vi "Write TDMS File.vi"(6 "Data Array":dbl[](array[numeric]), 8 "error in":errorcluster, 9 "Data & Time String":string, 10 "Header":string, 11 "Path":path) -> (0 "error out":errorcluster)   [LabVIEW 2009]
doc: "This subVI writes the object data to a file in a TDMS format. \n\nAAL 9/09"
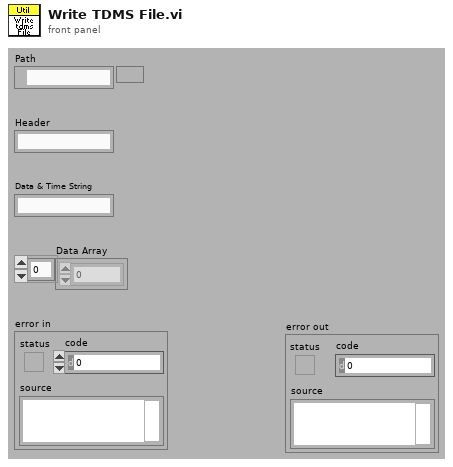
[diagram p1: front panel]
types:
  T1 = enum16{"open", "open or create", "create or replace", "create", "open (read-only)"}
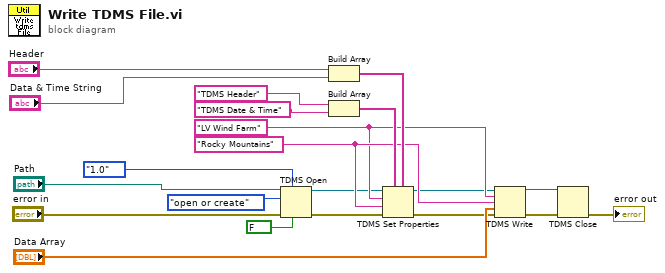
[diagram p0: block diagram]
diagram:
  w16 = "Rocky Mountains"
  w15 = "LV Wind Farm"
  n1 = TDMS Open(6:FALSE ("disable buffering (T)"), 7:enum16{"1.0", "2.0"}."1.0" ("file format version (2.0)"), 8:"error in", 10:T1."open or create" ("operation (0:open)"), 11:"Path") -> (0:w7:errorcluster, 3:w10:refnum<k34>)  [unwired: 1 in]
  n2 = Build Array("Header", "Data & Time String") -> (w21:string[])
  n3 = Build Array("TDMS Header", "TDMS Date & Time") -> (w20:string[])
  n4 = TDMS Set Properties(5:w21, 7:w20, 8:w7, 9:w16, 10:w15, 11:w10) -> (0:w8:errorcluster, 3:w11:refnum<k34>)  [unwired: 2 out]
  n5 = TDMS Write(0:w11, 5:w15, 7:w16, 9:"Data Array", 11:w8) -> (4:w12:refnum<k34>, 15:w9:errorcluster)  [unwired: 1 in, 2 out]
  n6 = TDMS Close(8:w9, 11:w12) -> (0:→"error out":errorcluster)
